vi "(SubVI)Ex and Force and fit .vi"(0 "QPD signal Out":dbl[](array[numeric]), 1 "Numeric":dbl, 7 "Position Array Out":dbl[](array[numeric]), 9 "control Cluster":T2={"laser power (mW)"=10.0, "center position shift (um)"=0.0001, "center QPD shift (V)"=0.0001, "Fc-cal-array"=[0.004414, 0.00367], "Convf-cal-array"=[0.19240621, 0.01244886], "Length offset"=400.0, "Force offset"=4.0, "trap height(nm)"=300.0, "bead radius(nm)"=515.0, "xDNA cut outside (nm)"=2000.0, "initial parameters"=[40.0, 1150.0], "fit only one side?"=FALSE, "T=positive (RHS)\nF=negative (LHS)"=FALSE, "Position Array Out"=[], "QPD signal Out"=[], "ci"=0.0, "yi"=0.0, "cr"=0.0, "yr"=0.0, "Force constant (pN/nm)"=0.0154, "conversion factor (V/um)"=2.6, "best fit parameters"=[], "best nonlinear fit"=[], "residue"=0.0, "Force-cut 2"=[], "xDNA-cut 2"=[]}, 12 "Numeric 2":dbl) -> (3 "xDNA-cut":dbl[](array[numeric]), 4 "best nonlinear fit":dbl[](array[numeric]), 6 "XY Graph 2":T3(graph), 8 "Force-cut":dbl[](array[numeric]), 10 "best fit parameters":dbl[](array[numeric]), 14 "output cluster":T1, 15 "error out":errorcluster)   [LabVIEW 2014]
uses:
  <vilib>/gmath/NI_Gmath.lvlib
  <vilib>/gmath/NumericalOptimization/Nonlinear Curve Fit LM formula string.vi
panel:
  # "Lp"
  # "L0"
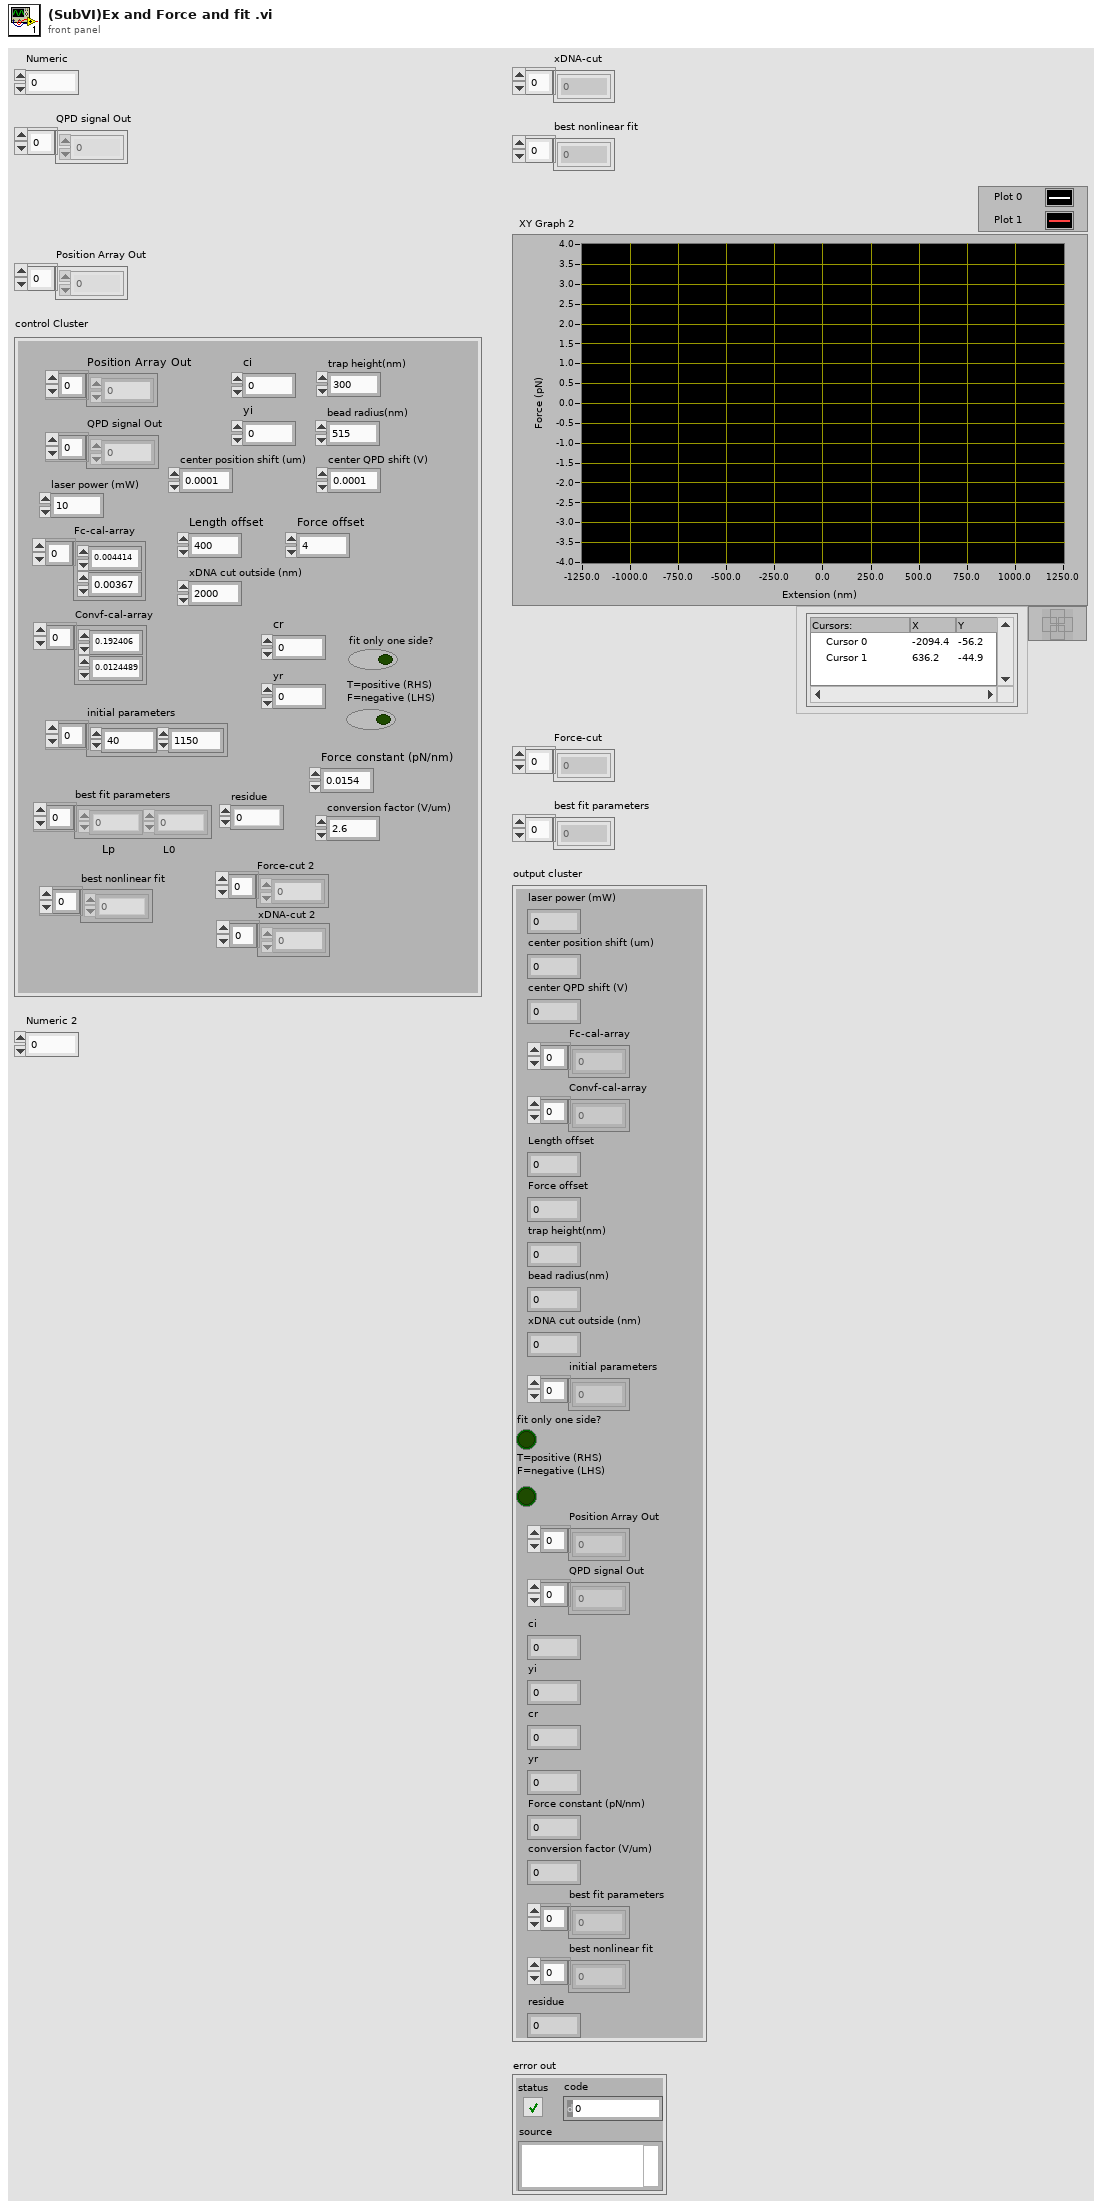
[diagram p1: front panel]
types:
  T1 = cluster{"laser power (mW)":dbl, "center position shift (um)":dbl, "center QPD shift (V)":dbl, "Fc-cal-array":dbl[], "Convf-cal-array":dbl[], "Length offset":dbl, "Force offset":dbl, "trap height(nm)":dbl, "bead radius(nm)":dbl, "xDNA cut outside (nm)":dbl, "initial parameters":dbl[], "fit only one side?":bool, "T=positive (RHS)\nF=negative (LHS)":bool, "Position Array Out":dbl[], "QPD signal Out":dbl[], "ci":dbl, "yi":dbl, "cr":dbl, "yr":dbl, "Force constant (pN/nm)":dbl, "conversion factor (V/um)":dbl, "best fit parameters":dbl[], "best nonlinear fit":dbl[], "residue":dbl}
  T2 = cluster{"laser power (mW)":dbl, "center position shift (um)":dbl, "center QPD shift (V)":dbl, "Fc-cal-array":dbl[], "Convf-cal-array":dbl[], "Length offset":dbl, "Force offset":dbl, "trap height(nm)":dbl, "bead radius(nm)":dbl, "xDNA cut outside (nm)":dbl, "initial parameters":dbl[], "fit only one side?":bool, "T=positive (RHS)\nF=negative (LHS)":bool, "Position Array Out":dbl[], "QPD signal Out":dbl[], "ci":dbl, "yi":dbl, "cr":dbl, "yr":dbl, "Force constant (pN/nm)":dbl, "conversion factor (V/um)":dbl, "best fit parameters":dbl[], "best nonlinear fit":dbl[], "residue":dbl, "Force-cut 2":dbl[], "xDNA-cut 2":dbl[]}
  T3 = cluster{"cut-full xDNA":dbl[], "cut-full Force":dbl[]}
  T4 = cluster{"model":string, "Parameters":string[], "x":string}
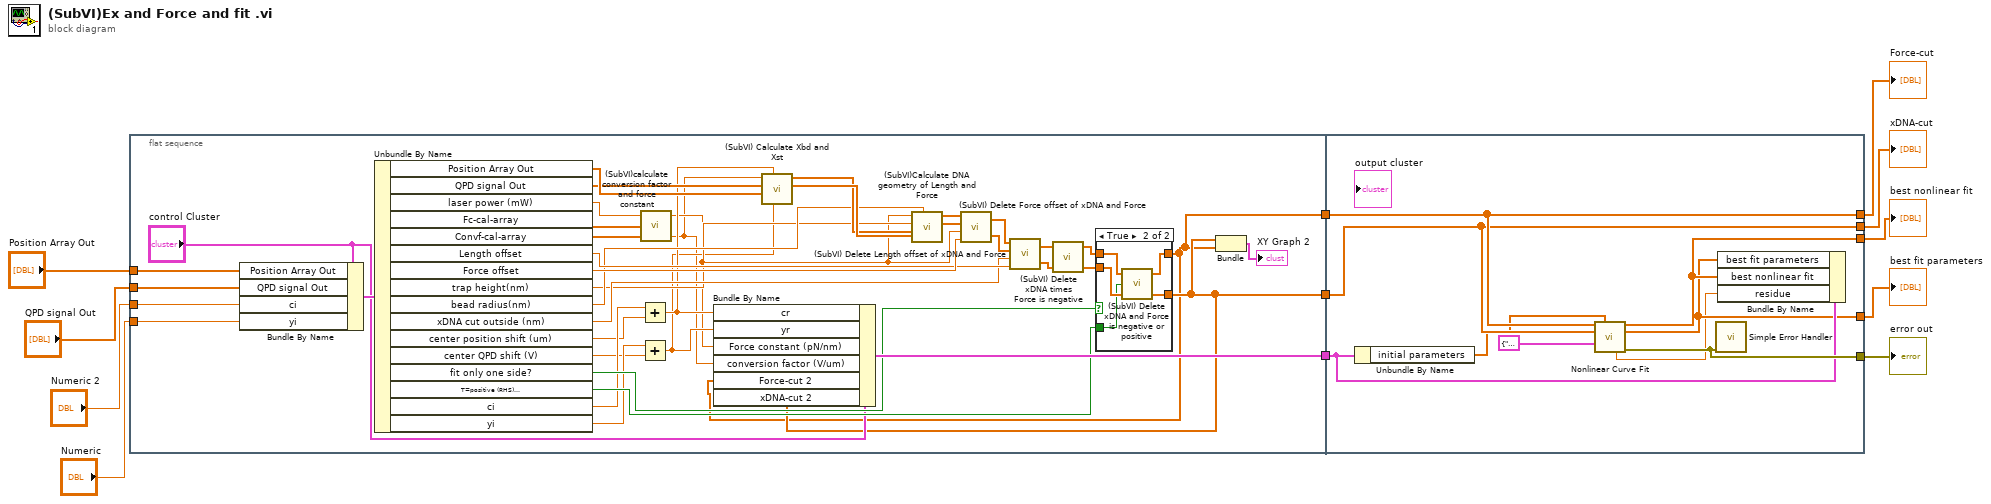
[diagram p0: block diagram]
diagram:
  n1 = flat-sequence {
    tunnel: [w13] -> w12
    tunnel: [w14] -> w11
    tunnel: [w52] -> w10
    tunnel: "Position Array Out" -> [w51]
    tunnel: "QPD signal Out" -> [w50]
    tunnel: "Numeric 2" -> [w49]
    tunnel: "Numeric" -> [w48]
    tunnel: [w66] -> w2
    tunnel: [w67] -> w1
    tunnel: w12 -> [w67]
    tunnel: w11 -> [w66]
    tunnel: [w65] -> w3
    tunnel: w10 -> [w63]
    tunnel: [w62] -> w4
    tunnel: [w61] -> w5
    frame #0 {
      n2 = Bundle By Name(cluster="control Cluster", "Position Array Out"=w51, "QPD signal Out"=w50, "ci"=w49, "yi"=w48) -> (w28:T2)
      n3 = Unbundle By Name(w28) -> ("Position Array Out"=w27:dbl[], "QPD signal Out"=w26:dbl[], "laser power (mW)"=w38:dbl, "Fc-cal-array"=w37:dbl[], "Convf-cal-array"=w36:dbl[], "Length offset"=w34:dbl, "Force offset"=w35:dbl, "trap height(nm)"=w31:dbl, "bead radius(nm)"=w32:dbl, "xDNA cut outside (nm)"=w33:dbl, "center position shift (um)"=w23:dbl, "center QPD shift (V)"=w22:dbl, "fit only one side?"=w30:bool, "T=positive (RHS)\nF=negative (LHS)"=w29:bool, "ci"=w25:dbl, "yi"=w24:dbl)
      n4 = Add(x=w25, y=w23) -> (x+y=w20:dbl)
      n5 = Add(x=w24, y=w22) -> (x+y=w19:dbl)
      n6 = call "(SubVI)calculate conversion factor and force constant.vi"("X=T\nY=F"=w36, 4:w37, "laser power (mW)"=w38) -> ("conversion factor (V/um)"=w17:dbl, "force constant (pN/nm)"=w18:dbl)  [unwired: 1 in]
      n7 = call "(SubVI) Calculate Xbd and Xst.vi"("yr"=w19, "cr"=w20, "Stage Position"=w27, "QPD signal"=w26, "conversion factor (V/um)"=w17) -> ("Xst"=w46:dbl[], "Xbd"=w45:dbl[])  [unwired: 5 in]
      n8 = call "(SubVI)Calculate DNA geometry of Length and Force.vi"("trap height(nm)"=w46, "bead radius(nm)"=w32, 9:w45, "Xst"=w31, "Xbd"=w18) -> ("xDNA"=w44:dbl[], "Force"=w43:dbl[])  [unwired: 4 in, 1 out]
      n9 = call "(SubVI) Delete Force offset of xDNA and Force.vi"("Force offset"=w35, "force constant"=w18, "xDNA"=w44, "Force"=w43) -> ("cut-full xDNA"=w41:dbl[], "cut-full Force"=w42:dbl[])
      n10 = call "(SubVI) Delete Length offset of xDNA and Force.vi"("Length offset"=w34, "xDNA cut outside (nm)"=w33, "xDNA"=w41, "Force"=w42) -> ("cut-full xDNA"=w39:dbl[], "cut-full Force"=w40:dbl[])
      n11 = call "(SubVI) Delete xDNA times Force is negative.vi"("xDNA"=w39, "Force"=w40) -> ("xDNA-cut"=w15:dbl[], "Force-cut"=w16:dbl[])  [unwired: 2 in]
      n12 = case shown="True" w30 {
        tunnel: w16 -> [w54 w59]
        tunnel: w15 -> [w53 w58]
        tunnel: [w53 w57] -> w14
        tunnel: [w54 w56] -> w13
        tunnel: w29 -> [_ w55]
        frame False {
        }
        frame True {
          n13 = call "(SubVI) Delete xDNA and Force is negative or positive.vi"("xDNA"=w58, "T=positive (RHS)\nF=negative (LHS)"=w55, "Force"=w59) -> ("xDNA-cut"=w57:dbl[], "Force-cut"=w56:dbl[])  [unwired: 1 in]
        }
      }
      n14 = Bundle By Name(cluster="control Cluster", "cr"=w20, "yr"=w19, "Force constant (pN/nm)"=w18, "conversion factor (V/um)"=w17, "Force-cut 2"=w13, "xDNA-cut 2"=w14) -> (w52:T2)
      n15 = Bundle("xDNA-cut"=w14, "Force-cut"=w13) -> (→"XY Graph 2":cluster{"xDNA-cut":dbl[], "Force-cut":dbl[]})  [unwired: 1 out]
    }
    frame #1 {
      n16 = Unbundle By Name(w63) -> ("initial parameters"=w64:dbl[])
      n17 = call-poly <vilib>:"Nonlinear Curve Fit.vi"("Y"=w67, "initial parameters"=w64, "X"=w66, "model description"=T4 {"model"="4.08687*(1/a1)*(sign(u)*1/4*(1-sign(u)*u/a2)^(-2)-(1/4*sign(u))+u/a2)", "Parameters"=["a1", "a2"], "x"="u"}) -> ("best nonlinear fit"=w62:dbl[], "best fit parameters"=w61:dbl[], "residue"=w60:dbl, "error out"=w65:errorcluster)  [unwired: 3 in, 5 out]
      n18 = call <vilib>:"Simple Error Handler.vi"("error in (no error)"=w65) -> ()  [unwired: 4 in, 5 out]
      n19 = Bundle By Name(cluster=w63, "best fit parameters"=w61, "best nonlinear fit"=w62, "residue"=w60) -> ()  [unwired: 1 out]
    }
  }
  "best fit parameters" <- w5
  "best nonlinear fit" <- w4
  "error out" <- w3
  "xDNA-cut" <- w2
  "Force-cut" <- w1
